vi "CarrierRx.vi"(9 "Phase":dbl, 10 "Carrier Frequency":dbl=10.1 caption="Frequency", 11 "Carrier Amplitude":dbl=1.0 caption="Amplitude") -> (2 "I(t) Carrier":waveform(dbl), 3 "R(t) Carrier":waveform(dbl))   [LabVIEW 2014]
uses:
  <vilib>/Analysis/NI_AALPro.lvlib
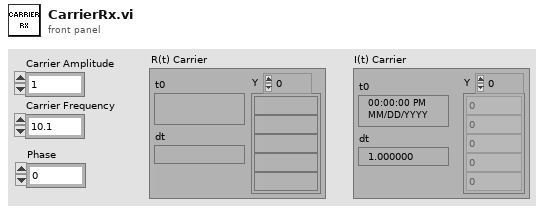
[diagram p1: front panel]
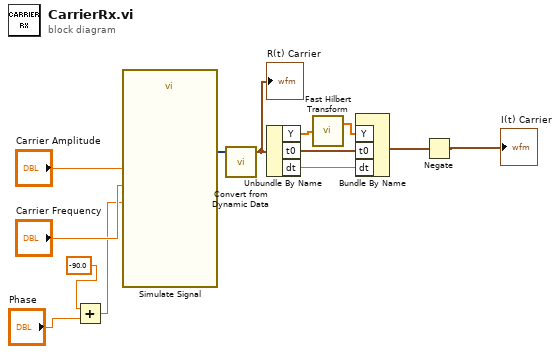
[diagram p0: block diagram]
diagram:
  n1 = Add(x=-90.0 ("Phase"), y="Phase") -> (x+y=w1:dbl)
  n2 = call "Simulate Signal"("Frequency"="Carrier Frequency", "Amplitude"="Carrier Amplitude", "Phase"=w1) -> ("Sine"=w11:dynamicdata)  [unwired: 11 in, 1 out]
  n3 = call "Convert from Dynamic Data"("Dynamic Data Type"=w11) -> ("Waveform"=w6:waveform(dbl))  [unwired: 3 in]
  "R(t) Carrier" <- w6
  n4 = Unbundle By Name(w6) -> ("Y"=w10:dbl[], "t0"=w9:timestamp, "dt"=w8:dbl)
  n5 = call <vilib>:"Fast Hilbert Transform.vi"("X"=w10) -> ("Hilbert{X}"=w7:dbl[])  [unwired: 1 out]
  n6 = Bundle By Name("Y"=w7, "t0"=w9, "dt"=w8) -> (w4:waveform(dbl))  [unwired: 1 in]
  n7 = Negate(x=w4) -> (-x=→"I(t) Carrier":waveform(dbl))
